vi "InitDevice.vi"(6 "DevInd":u32, 7 "ID(Hex 高位有效)":string="312", 8 "错误输入":errorcluster caption="错误输入（无错误）", 9 "InitConfig":T2={"AccCode"=0, "AccMask"=4294967295, "Reserved"=0, "Filter"=0, "kCanBaud"=12, "Timing0"=10, "Timing1"=0, "Mode"=0, "CanRx_IER"=1} {"CanRx_IER" items=["0", "1"]; "kCanBaud" items=["250k bps"=10, "10k bps"=2, "5k bps"=1, "50k bps"=5, "40k bps"=4, "20k bps"=3, "80k bps"=6, "100k bps"=7, "125k bps"=8, "200k bps"=9, "400k bps"=11, "500k bps"=12, "666k bps"=13, "800k bps"=14, "1000k bps"=15]; "Mode" items=["Normal", "Self TX-RX"]; "Filter" items=["Single Filter", "Dual Filter"]; "AccCode" format="%08x"; "AccMask" format="%08x"; "Timing0" format="%02x"; "Timing1" format="%02x"}, 10 "CanChannel":u32, 11 "DeviceType":T1=3 items=["PCI-CAN200"=7, "USB-CAN"=2, "USB-CAN200"=3]) -> (0 "错误输出":errorcluster, 1 "DevIndex":u32, 2 "Result":bool, 3 "DeviceTypeOut":T1=3 items=["PCI-CAN200"=7, "USB-CAN"=2, "USB-CAN200"=3], 4 "CanIndex":u32)   [LabVIEW 2013]
uses:
  InitConfig.ctl
  DevType.ctl
  VCI_CAN.dll
panel:
  in  "滤波":bool=TRUE
  out "输出簇":T2={"AccCode"=0, "AccMask"=4294967295, "Reserved"=0, "Filter"=0, "kCanBaud"=10, "Timing0"=0, "Timing1"=0, "Mode"=0, "CanRx_IER"=0} {"CanRx_IER" items=["0", "1"]; "kCanBaud" items=["250k bps"=10, "10k bps"=2, "5k bps"=1, "50k bps"=5, "40k bps"=4, "20k bps"=3, "80k bps"=6, "100k bps"=7, "125k bps"=8, "200k bps"=9, "400k bps"=11, "500k bps"=12, "666k bps"=13, "800k bps"=14, "1000k bps"=15]; "Mode" items=["Normal", "Self TX-RX"]; "Filter" items=["Single Filter", "Dual Filter"]; "AccCode" format="%08x"; "AccMask" format="%08x"; "Timing0" format="%02x"; "Timing1" format="%02x"}
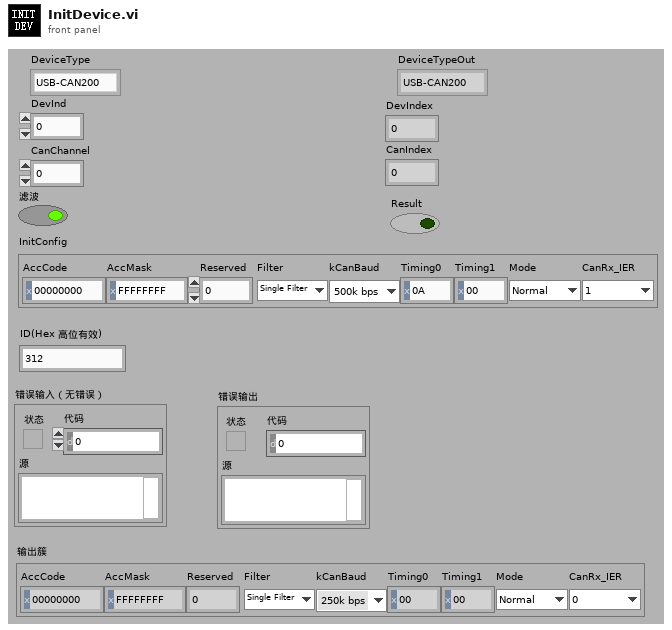
[diagram p1: front panel]
types:
  T1 = typedef "DevType.ctl" = u16
  T2 = typedef "InitConfig.ctl" = cluster{"AccCode":u32, "AccMask":u32, "Reserved":u32, "Filter":u8, "kCanBaud":u8, "Timing0":u8, "Timing1":u8, "Mode":u8, "CanRx_IER":u8}
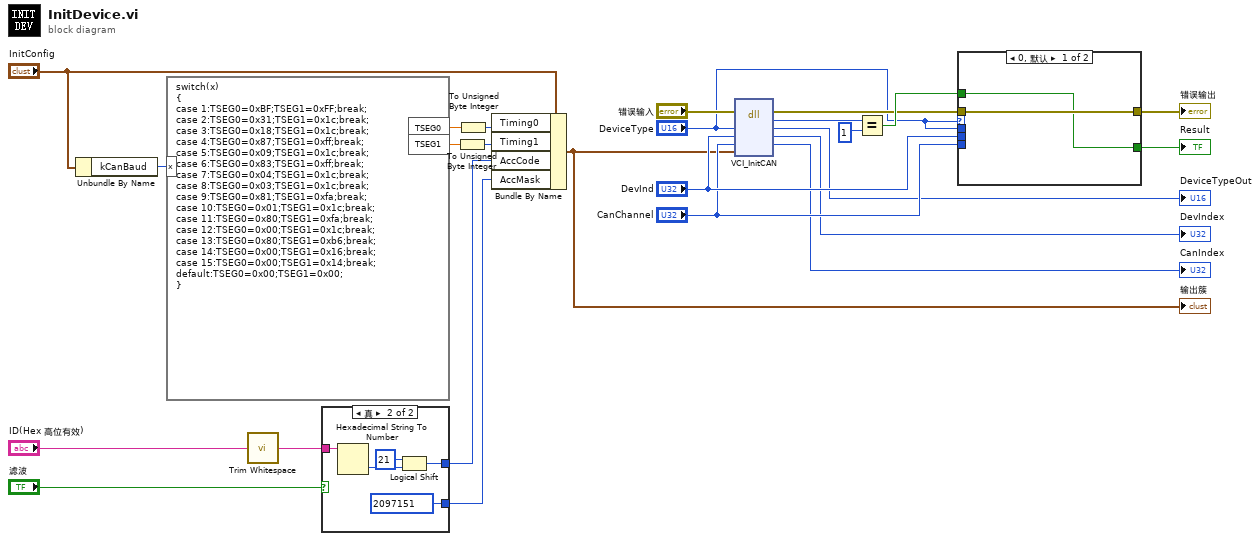
[diagram p0: block diagram]
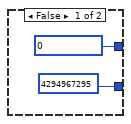
[diagram p2: hidden frame]
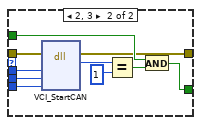
[diagram p3: hidden frame]
diagram:
  n1 = Unbundle By Name("InitConfig") -> ("kCanBaud"=w22:u8)
  n2 = formula code="switch(x)\n{ \ncase 1:TSEG0=0xBF;TSEG1=0xFF;break;\ncase 2:TSEG0=0x31;TSEG1=0x1c;break;\ncase 3:TSEG0=0x18;TSEG1=0x1c;break;\ncase 4:TSEG0=0x87;TSEG1=0xff;break;\ncase 5:TSEG0=0x09;TSEG1=0x1c;break;\ncase 6:TSEG0=0x83;TSEG1=0xff;break;\ncase 7:TSEG0=0x04;TSEG1=0x1c;break;\ncase 8:TSEG0=0x03;TSEG1=0x1c;break;\ncase 9:TSEG0=0x81;TSEG1=0xfa;break;\ncase 10:TSEG0=0x01;TSEG1=0x1c;break;\ncase 11:TSEG0=0x80;TSEG1=0xfa;break;\ncase 12:TSEG0=0x00;TSEG1=0x1c;break;\ncase 13:TSEG0=0x80;TSEG1=0xb6;break;\ncase 14:TSEG0=0x00;TSEG1=0x16;break;\ncase 15:TSEG0=0x00;TSEG1=0x14;break;\ndefault:TSEG0=0x00;TSEG1=0x00;\n}"("x"=w22) -> ("TSEG0"=w20:dbl, "TSEG1"=w21:dbl)
  n3 = call <vilib>:"Trim Whitespace.vi"("string"="ID(Hex 高位有效)") -> ("trimmed string"=w7:string)  [unwired: 1 in]
  n4 = case shown="真" "滤波" {
    tunnel: w7 -> [_ w31]
    tunnel: [u32 0 ("验收码") w28] -> w4
    tunnel: [u32 4294967295 ("屏蔽码") u32 2097151 ("屏蔽码")] -> w5
    frame False {
    }
    frame True {
      n5 = Hexadecimal String To Number(string=w31) -> (number=w29:u32)  [unwired: 2 in, 1 out]
      n6 = Logical Shift(y=i8 21, x=w29) -> (x << y=w28:u32)
    }
  }
  n7 = To Unsigned Byte Integer(number=w21) -> (unsigned 8bit integer=w18:u8)
  n8 = To Unsigned Byte Integer(number=w20) -> (unsigned 8bit integer=w19:u8)
  n9 = Bundle By Name(cluster="InitConfig", "Timing0"=w19, "Timing1"=w18, "AccCode"=w4, "AccMask"=w5) -> (w9:T2)
  "输出簇" <- w9
  n10 = dll-call lib="C:/Users/Administrator/Desktop/CAN/USBCAN/VCI_CAN.dll" fn="VCI_InitCAN"(error in="错误输入", "DevType"="DeviceType", "DevIndex"="DevInd", "CanIndex"="CanChannel", "pInitConfig"=w9) -> (error out=w12:errorcluster, "返回类型"=w24:u32, "DevType"=→"DeviceTypeOut":u32, "DevIndex"=→"DevIndex":u32, "CanIndex"=→"CanIndex":u32)  [unwired: 3 in, 1 out]
  n11 = Equal?(x=w24, y=u32 1) -> (x = y?=w14:bool)
  n12 = case shown="0, 默认" "DeviceType" {
    tunnel: "DeviceType" -> [_ w44]
    tunnel: "DevInd" -> [_ w43]
    tunnel: "CanChannel" -> [_ w42]
    tunnel: w14 -> [w33 w39]
    tunnel: [w33 w37] -> w13
    tunnel: w12 -> [w34 w36]
    tunnel: [w34 w35] -> w11
    frame 0, Default {
    }
    frame 2, 3 {
      n13 = dll-call lib="C:/Users/Administrator/Desktop/CAN/USBCAN/VCI_CAN.dll" fn="VCI_StartCAN"(error in=w36, "DeviceType"=w44, "DeciceInd"=w43, "CANInd"=w42) -> (error out=w35:errorcluster, "返回类型"=w41:u32)  [unwired: 5 in, 1 out]
      n14 = Equal?(x=w41, y=u32 1) -> (x = y?=w38:bool)
      n15 = And(x=w39, y=w38) -> (x .and. y?=w37:bool)
    }
  }
  "错误输出" <- w11
  "Result" <- w13
